vi "TDMS to Variant.vi"() -> ()   [LabVIEW 2021]
uses:
  Breeeze Utilities/UI/Tree Data Selector/Tree Data Selector.lvclass
  Breeeze Utilities/Breeze Utilities.lvlib
panel:
  out "Variant Path":string
  out "Tree Value":string
  out "Variant out":variant
  in  "Tree":string(tree)
  out "group names":string[](array[string])
  in  "File Path Control":path=path "\\\\Mac\\Home/Documents/Non-SCC/EMA/ATP 20220622 140935.tdms"
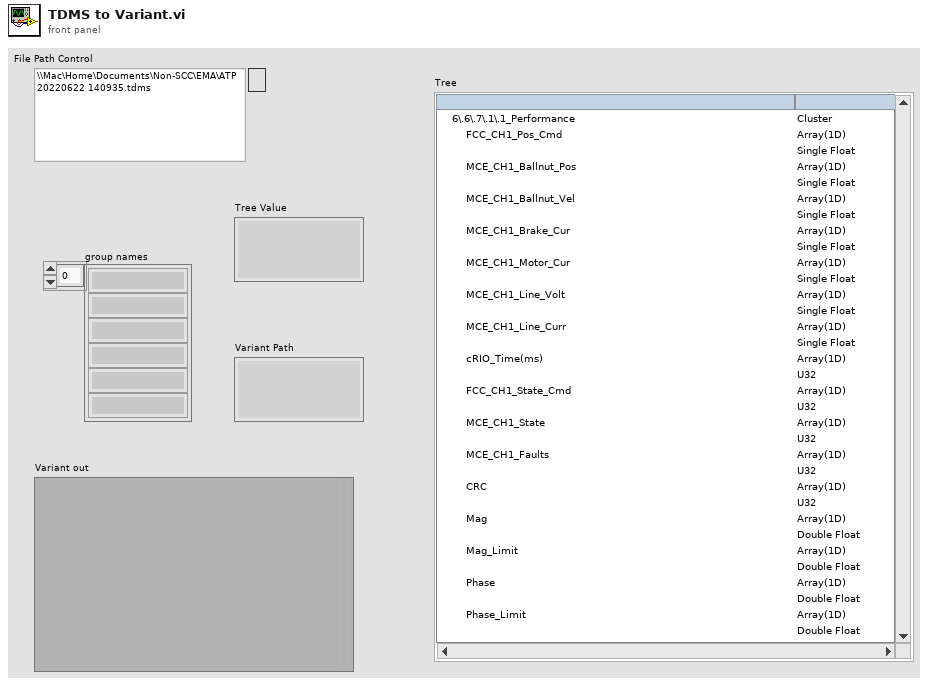
[diagram p1: front panel]
types:
  T1 = enum16{"open", "open or create", "create or replace", "create", "open (read-only)"}
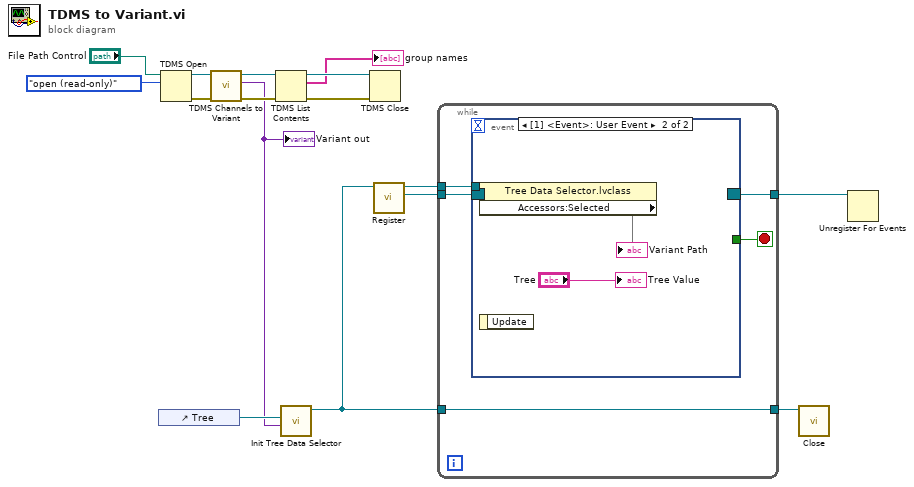
[diagram p0: block diagram]
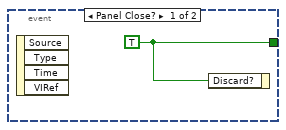
[diagram p2: hidden frame]
diagram:
  n1 = control-ref of="Tree"() -> (w11:refnum<vi>)
  n2 = TDMS Open(10:T1."open (read-only)" ("operation (0:open)"), 11:"File Path Control") -> (0:w5:errorcluster, 3:w6:refnum<k34>)  [unwired: 5 in]
  n3 = call "TDMS Channels to Variant.vi"("error in (no error)"=w5, "TDMS"=w6) -> ("error out"=w4:errorcluster, "Variant out"=w2:variant, "tdms file out"=w3:refnum<k34>)  [unwired: 7 in]
  "Variant out" <- w2
  n4 = TDMS List Contents(4:w4, 7:w3) -> (0:w13:errorcluster, 2:→"group names":string[], 3:w14:refnum<k34>)  [unwired: 1 in, 1 out]
  n5 = call "Init Tree Data Selector.vi"("Variant"=w2, "Tree Refnum"=w11) -> ("Tree Data Selector out"=w8:refnum<class "Tree Data Selector.lvclass">)  [unwired: 8 in, 1 out]
  n6 = TDMS Close(8:w13, 11:w14) -> ()  [unwired: 2 out]
  n7 = call "Register.vi"("Ref"=w8) -> ("Event"=w7:refnum<event-registration>, "Ref (Dup)"=w1:refnum<class "Tree Data Selector.lvclass">)  [unwired: 9 in]
  n8 = while {
    tunnel: w8 -> [w21]
    tunnel: [w21] -> w10
    tunnel: [w19] -> w9
    tunnel: w7 -> [w18]
    tunnel: w1 -> [w17]
    stop <- w20 stop-if-true
    n9 = event shown="[1] <Event>: User Event" {
      selector: w18 -> [_ _]
      dyn-events: [_ _] -> w19
      timeout: _ -> [_ _]
      tunnel: [w22 _] -> w20
      tunnel: w17 -> [_ w25]
      event Panel Close? {
        w22 = TRUE
        n10 = event-data() -> ()  [unwired: 1 in, 4 out]
        n11 = event-data("Discard?"=w22) -> ()  [unwired: 1 in, 1 out]
      }
      event User Event {
        n12 = property class="Tree Data Selector.lvclass"(reference=w25) -> ("Accessors:Selected"=→"Variant Path")  [unwired: 1 in, 2 out]
        n13 = event-data() -> ()  [unwired: 1 in, 1 out]
        "Tree Value" <- "Tree"
      }
    }
  }
  n14 = call-dynamic "Close.vi"("Tree Data Selector in"=w10) -> ()  [unwired: 10 in, 1 out]
  n15 = Unregister For Events(event registration refnum=w9) -> ()  [unwired: 1 in, 1 out]
